vi "CRYCalc Standard Error.vi"(4 "N(Samples #)":dbl=1000.0 min=1.0, 6 "Fs":dbl=1000.0 min=1.0, 8 "Harmonic RMS(V)":dbl[](array[numeric]), 9 "Harmonic Frequency":dbl[](array[numeric]), 10 "Power Spectrum(V^2)":dbl[](array[numeric]), 11 "X(t)":dbl[](array[numeric])) -> ()   [LabVIEW 2013]
uses:
  <vilib>/Analysis/2dsp.llb/Zero Padder (DBL).vi
  <vilib>/Analysis/NI_AALPro.lvlib
panel:
  out "size(s)":i32
  out "Zero size":i32
  out "In size":i32
  out "Waveform Graph 3":dbl[](graph)
  out "Waveform Graph 2":T1(graph)
  in  "Window":u16
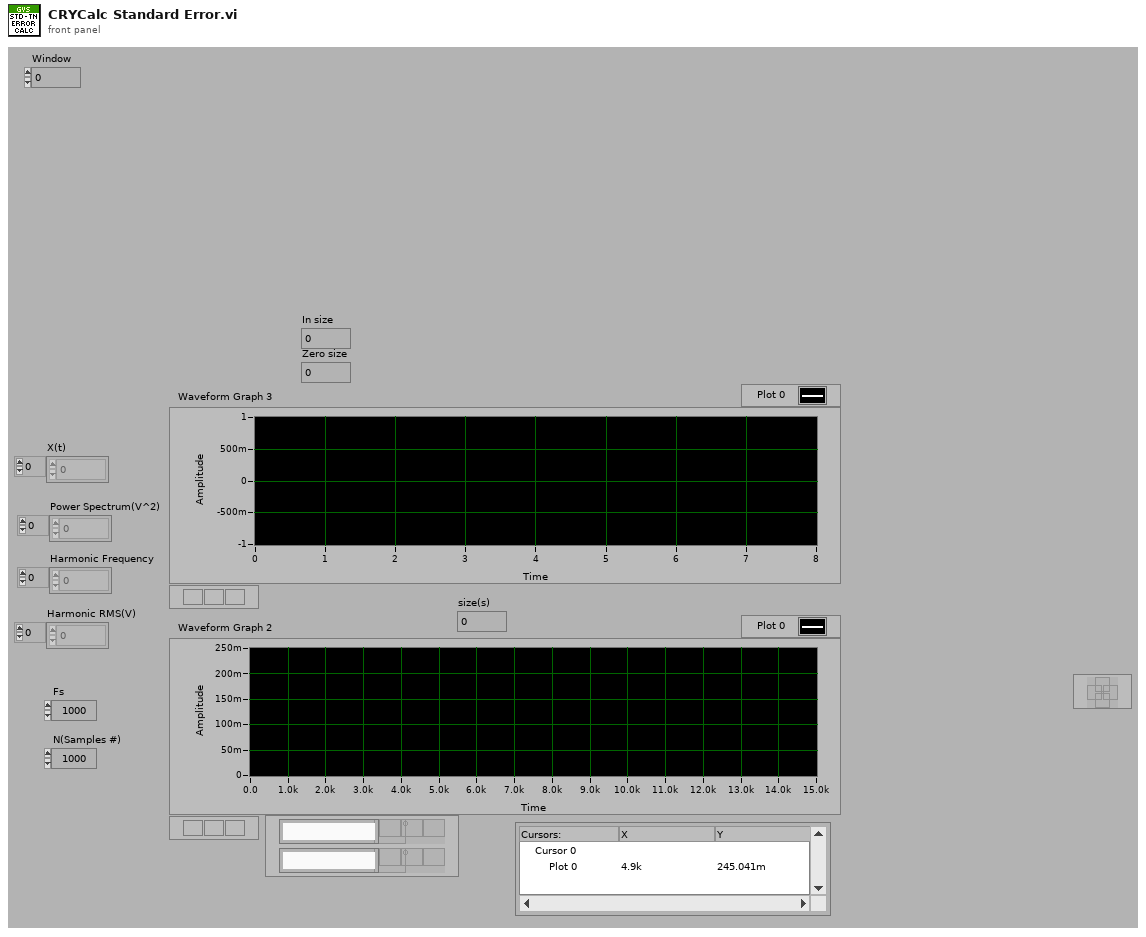
[diagram p1: front panel]
types:
  T1 = cluster{"x":dbl, dbl, "Power Spectrum (V^2 rms)":dbl[]}
  T2 = cluster{"x":dbl, "df":dbl, "Power Spectrum (V^2 rms)":dbl[]}
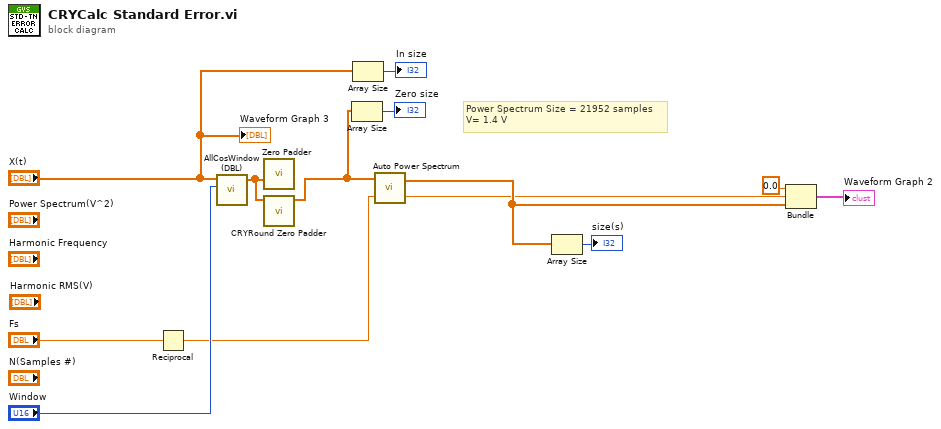
[diagram p0: block diagram]
diagram:
  # "Power Spectrum Size = 21952 samples\nV= 1.4 V"
  n1 = Reciprocal(x="Fs") -> (1/x=w4:dbl)
  n2 = call <vilib>:"AllCosWindow (DBL).vi"("window"="Window", "X"="X(t)") -> ("Windowed X"=w8:dbl[])  [unwired: 1 in, 3 out]
  n3 = call-poly <vilib>:"Zero Padder.vi"("Input Array"=w8) -> ()  [unwired: 1 in, 10 out]
  n4 = call "CRYRound Zero Padder.vi"("Vector in"=w8) -> ("Zero Padder Vector out"=w7:dbl[])  [unwired: 9 in, 1 out]
  n5 = Array Size(array=w7) -> (size(s)=→"Zero size":i32)
  n6 = Array Size(array="X(t)") -> (size(s)=→"In size":i32)
  n7 = call <vilib>:"Auto Power Spectrum.vi"("dt"=w4, "Signal (V)"=w7) -> ("df"=w1:dbl, "Power Spectrum (V^2 rms)"=w6:dbl[])
  n8 = Array Size(array=w6) -> (size(s)=→"size(s)":i32)
  n9 = Bundle("x"=0.0, "df"=w1, "Power Spectrum (V^2 rms)"=w6) -> (→"Waveform Graph 2":T2)  [unwired: 1 in]
  "Waveform Graph 3" <- "X(t)"
